vi "Polls.Compile.vi"(8 "error in (no error)":errorcluster, 11 "Section Ref in":T6 format="%.0x") -> (0 "error out":errorcluster, 1 "Poll Settings":T1[](array[typedef]), 2 "Service Channels":T3[](array[typedef]) {"Signal.Cmd.Refs"."Signal Refs" format="%.0x"; "Signal.Cmd.Info"."Signals"."Byte Order" items=["Little Endian", "Big Endian"]; "Signal.Cmd.Info"."Signals"."Data Type" items=["Signed", "Unsigned", "IEEE Float"]; "Settings.Refs"."Signal Refs" format="%.0x"; "Signal.Resp.Refs"."Signal Refs" format="%.0x"; "Signal.Resp.Info"."Signals"."Byte Order" items=["Little Endian", "Big Endian"]; "Signal.Resp.Info"."Signals"."Data Type" items=["Signed", "Unsigned", "IEEE Float"]; "Trigger.Refs"."Signal Refs" format="%.0x"; "Status.Refs"."Signal Refs" format="%.0x"}, 3 "Section Ref out":T6 format="%.0x")   [LabVIEW 2019, in "Diagnostics Addon System Explorer.lvlib"]
uses:
  Diagnostics Addon System Explorer.lvlib
  <vilib>/NI VeriStand/Custom Device API/Custom Device Item Ref.ctl
  Types/Service.Export.ctl
  Types/Frame.Ref.ctl
  Shared/Types/Type.ctl
  Shared/Types/Frame.Compile.ctl
  Shared/Types/Signal.ctl
  Shared/Types/Poll.Compiled.ctl
  Shared/Types/DPID.Rate.ctl
  Types/FG.Action.ctl
  Shared/SubVIs/Constants.vi
  <vilib>/NI VeriStand/Custom Device Tools/Custom Device Utility Library/NI VeriStand - Search for All Items by GUID.vi
  <vilib>/NI VeriStand/Custom Device Tools/Custom Device Utility Library/NI VeriStand - Search for Item by GUID.vi
  <vilib>/NI VeriStand/Custom Device API/NI VeriStand - Get Item Children.vi
  <vilib>/NI VeriStand/Custom Device Tools/Custom Device Utility Library/NI VeriStand - Search for Item by Name.vi
  <vilib>/NI/NI VeriStand Advanced SysDef API/SysDef API/SysDef.Property.Set.vi
  <vilib>/NI/NI VeriStand Advanced SysDef API/_SubVIs/SysDef.Property.Set.U32.vi
  <vilib>/NI VeriStand/Custom Device API/NI VeriStand - Get Item Property.vi
  <vilib>/NI VeriStand/Custom Device API/Get Item Property (U32).vi
  <vilib>/NI VeriStand/Custom Device Tools/Custom Device Utility Library/Custom Device Utility Library.lvlib
  <vilib>/NI VeriStand/Custom Device API/Custom Device API.lvlib
  Shared/Diagnostics Addon Shared.lvlib
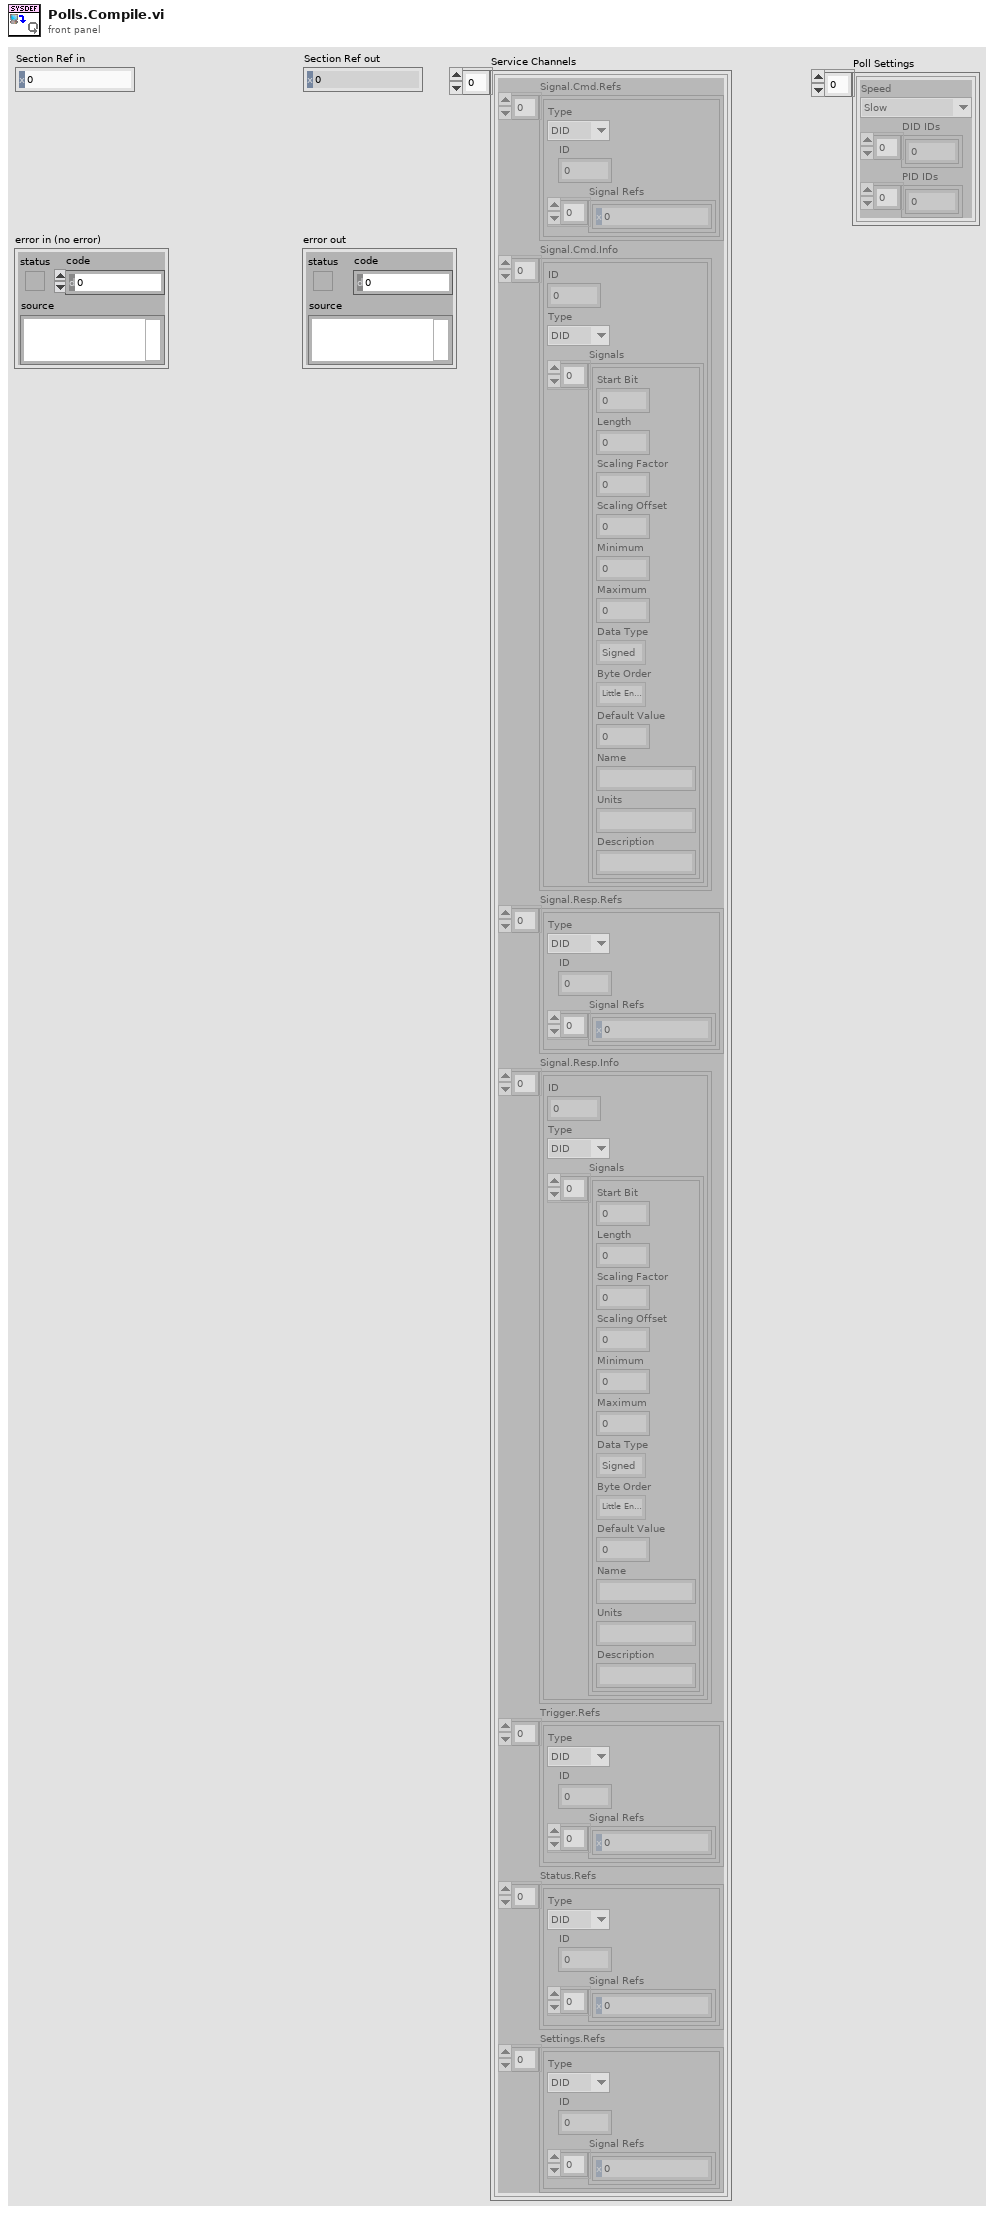
[diagram p1: front panel]
types:
  T1 = typedef "Diagnostics Addon Shared.lvlib/Poll.Compiled.ctl" = cluster{"Speed":T2, "DID IDs":u32[], "PID IDs":u32[]}
  T2 = typedef "Diagnostics Addon Shared.lvlib/DPID.Rate.ctl" = enum16{"Slow", "Medium", "Fast"}
  T3 = typedef "Diagnostics Addon System Explorer.lvlib/Service.Export.ctl" = cluster{"Signal.Cmd.Refs":T4[], "Signal.Cmd.Info":T7[], "Signal.Resp.Refs":T4[], "Signal.Resp.Info":T7[], "Trigger.Refs":T4[], "Status.Refs":T4[], "Settings.Refs":T4[]}
  T4 = typedef "Diagnostics Addon System Explorer.lvlib/Frame.Ref.ctl" = cluster{"Type":T5, "ID":u32, "Signal Refs":T6[]}
  T5 = typedef "Diagnostics Addon Shared.lvlib/Type.ctl" = enum16{"DID", "CDID", "PID", "CPID", "Read Memory", "Write Memory", "IO Control", "Routine Start", "Routine Request", "Routine Stop", "User Defined", "DTC Control", "Clear DTCs", "Read DTCs", "Start DTCs", "DTC Change Count", "Tester Present", "Unlock ECU", "Reset ECU", "Diag Session Control", "Communication Control", "Configure DPIDs", "Start DPIDs", "Stop DPIDs", "Poll Control", "Diag CAN Control"}
  T6 = typedef "Custom Device API.lvlib/Custom Device Item Ref.ctl" = u64
  T7 = typedef "Diagnostics Addon Shared.lvlib/Frame.Compile.ctl" = cluster{"ID":u32, "Type":T5, "Signals":T8[]}
  T8 = typedef "Diagnostics Addon Shared.lvlib/Signal.ctl" = cluster{"Start Bit":u32, "Length":u32, "Scaling Factor":dbl, "Scaling Offset":dbl, "Minimum":dbl, "Maximum":dbl, "Data Type":u32, "Byte Order":u32, "Default Value":dbl, "Name":string, "Units":string, "Description":string}
  T9 = typedef "Diagnostics Addon System Explorer.lvlib/FG.Action.ctl" = enum16{"Get", "Set"}
  T10 = typedef "Diagnostics Addon System Explorer.lvlib/Poll.Settings.ctl" = cluster{"Input Channels":T11[], "Speed":T2}
  T11 = typedef "Diagnostics Addon System Explorer.lvlib/Poll.LinkedNode.ctl" = cluster{"Node ID":u64}
  T12 = typedef "Custom Device API.lvlib/Custom Device Item Info.ctl" = cluster{"Name":string, "Is Channel":bool, "GUID":string, "Is Waveform":bool}
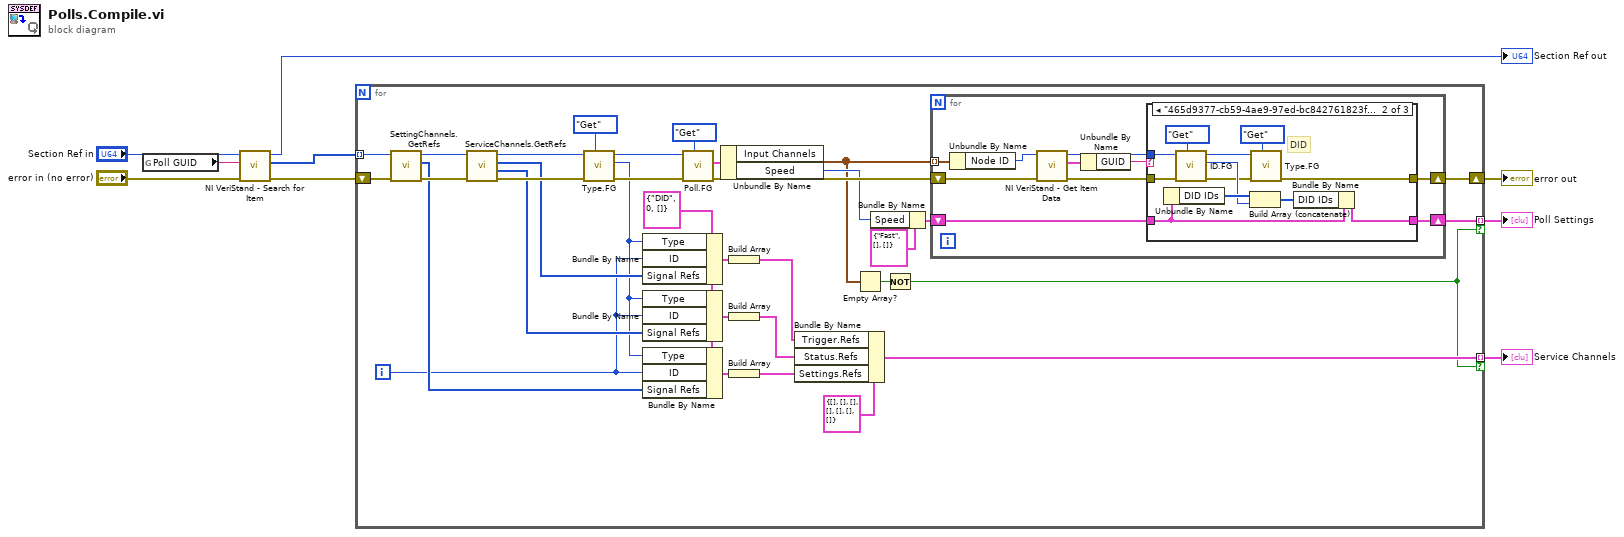
[diagram p0: block diagram]
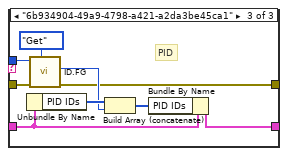
[diagram p3: hidden frame]
diagram:
  n1 = global read "Constants.vi" "Poll GUID"() -> (w9:string)
  n2 = call-poly <vilib>:"NI VeriStand - Search for Item.vi"("error in"="error in (no error)", "Item GUID"=w9, "Section Ref in"="Section Ref in") -> ("error out"=w8:errorcluster, "Item Refs"=w7:T6[], "Section Ref out"=→"Section Ref out":T6)  [unwired: 5 in, 1 out]
  n3 = for {
    tunnel: w7 -> [w11] mode=indexing
    shift-right: [w37] -> w4
    shift-left: w8 -> [w35]
    tunnel: [w38] -> w1 mode=indexing if=w13
    tunnel: [w14] -> w2 mode=indexing if=w13
    i -> [w10]
    w24 = T4 {"Type"=enum."DID", "ID"=0, "Signal Refs"=[]} ("cluster")
    n4 = call "SettingChannels.GetRefs.vi"("error in (no error)"=w35, "Item Ref in"=w11) -> ("error out"=w31:errorcluster, "Settings"=w21:T6[], "Section Ref out"=w30:T6)  [unwired: 7 in]
    n5 = call "ServiceChannels.GetRefs.vi"("error in (no error)"=w31, "Item Ref in"=w30) -> ("error out"=w29:errorcluster, "Status"=w22:T6[], "Trigger"=w23:T6[], "Section Ref out"=w28:T6)  [unwired: 6 in]
    n6 = call "Type.FG.vi"("Action"=FG.Action."Get", "error in (no error)"=w29, "Device Item Ref in"=w28) -> ("error out"=w34:errorcluster, "Type"=w17:T5, "Device Item Ref out"=w12:T6)  [unwired: 6 in]
    n7 = Bundle By Name(cluster=w24, "Type"=w17, "ID"=w10, "Signal Refs"=w23) -> (w27:T4)
    n8 = Bundle By Name(cluster=w24, "Type"=w17, "ID"=w10, "Signal Refs"=w22) -> (w26:T4)
    n9 = Bundle By Name(cluster=w24, "Type"=w17, "ID"=w10, "Signal Refs"=w21) -> (w25:T4)
    n10 = call "Poll.FG.vi"("Action"=FG.Action."Get", "error in"=w34, "Parent Ref"=w12) -> ("error out"=w40:errorcluster, "Selected Channels out"=w41:T10)  [unwired: 6 in, 1 out]
    n11 = Unbundle By Name(w41) -> ("Input Channels"=w16:T11[], "Speed"=w36:T2)
    n12 = Build Array(w27) -> (w20:T4[])
    n13 = Build Array(w26) -> (w19:T4[])
    n14 = Build Array(w25) -> (w18:T4[])
    n15 = Bundle By Name(cluster=T3 {"Signal.Cmd.Refs"=[], "Signal.Cmd.Info"=[], "Signal.Resp.Refs"=[], "Signal.Resp.Info"=[], "Trigger.Refs"=[], "Status.Refs"=[], "Settings.Refs"=[]}, "Trigger.Refs"=w20, "Status.Refs"=w19, "Settings.Refs"=w18) -> (w14:T3)
    n16 = Empty Array?(array=w16) -> (empty?=w15:bool)
    n17 = Bundle By Name(cluster=T1 {"Speed"=enum."Fast", "DID IDs"=[], "PID IDs"=[]}, "Speed"=w36) -> (w39:T1)
    n18 = Not(x=w15) -> (.not. x?=w13:bool)
    n19 = for {
      tunnel: w16 -> [w53] mode=indexing
      shift-right: [w46] -> w37
      shift-left: w40 -> [w51]
      shift-right: [w45] -> w38
      shift-left: w39 -> [w47]
      n20 = Unbundle By Name(w53) -> ("Node ID"=w50:u64)
      n21 = call <vilib>:"NI VeriStand - Get Item Data.vi"("error in (no error)"=w51, "Item Ref in"=w50) -> ("error out"=w48:errorcluster, "Item Info"=w52:T12, "Item Ref out"=w44:T6)  [unwired: 6 in, 1 out]
      n22 = Unbundle By Name(w52) -> ("GUID"=w49:string)
      n23 = case shown="\"465d9377-cb59-4ae9-97ed-bc842761823f\"" w49 {
        tunnel: w48 -> [w55 w66 w75]
        tunnel: w47 -> [w54 w65 w72]
        tunnel: [w55 w57 w69] -> w46
        tunnel: [w54 w60 w68] -> w45
        tunnel: w44 -> [_ w62 w71]
        frame Default {
        }
        frame "465d9377-cb59-4ae9-97ed-bc842761823f" {
          # "DID"
          n24 = Unbundle By Name(w65) -> ("DID IDs"=w64:u32[])
          n25 = call "ID.FG.vi"("Action"=FG.Action."Get", "error in (no error)"=w66, "Device Item Ref in"=w62) -> ("error out"=w58:errorcluster, "ID"=w63:u32, "Device Item Ref out"=w56:T6)  [unwired: 6 in]
          n26 = Build Array (concatenate)(w64, w63) -> (w61:u32[])
          n27 = call "Type.FG.vi"("Action"=FG.Action."Get", "error in (no error)"=w58, "Device Item Ref in"=w56) -> ("error out"=w57:errorcluster)  [unwired: 6 in, 2 out]
          n28 = Bundle By Name(cluster=w65, "DID IDs"=w61) -> (w60:T1)
        }
        frame "6b934904-49a9-4798-a421-a2da3be45ca1" {
          # "PID"
          n29 = Unbundle By Name(w72) -> ("PID IDs"=w74:u32[])
          n30 = call "ID.FG.vi"("Action"=FG.Action."Get", "error in (no error)"=w75, "Device Item Ref in"=w71) -> ("error out"=w69:errorcluster, "ID"=w70:u32)  [unwired: 6 in, 1 out]
          n31 = Build Array (concatenate)(w74, w70) -> (w73:u32[])
          n32 = Bundle By Name(cluster=w72, "PID IDs"=w73) -> (w68:T1)
        }
      }
    }
  }
  "error out" <- w4
  "Service Channels" <- w2
  "Poll Settings" <- w1
